vi "Resize Message String & Dialog Window.vi"(6 "Max Number of Lines":i32, 8 "Error In":errorcluster, 9 "Message":string, 10 "Controls & Indicators":T1, 11 "VI Refnum":refnum<vi>) -> (0 "Error Out":errorcluster, 3 "VI Refnum out":refnum<vi>)   [LabVIEW 2021, in "GUI.lvlib"]
uses:
  GUI.lvlib
  Error/Error.lvlib
  Buttons/Buttons.lvlib
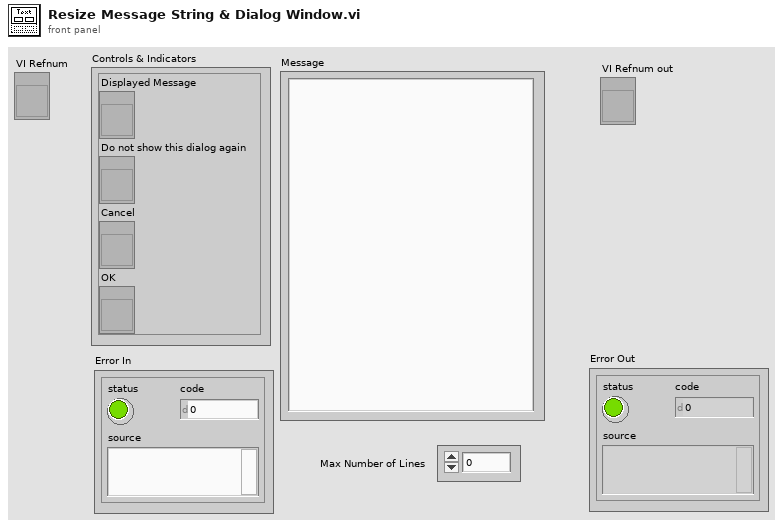
[diagram p1: front panel]
types:
  T1 = cluster{"Displayed Message":refnum<vi>, "Do not show this dialog again":refnum<vi>, "Cancel":refnum<vi>, "OK":refnum<vi>}
  T2 = typedef "LVRectTypeDef.ctl" = cluster{"Left":i16, "Top":i16, "Right":i16, "Bottom":i16}
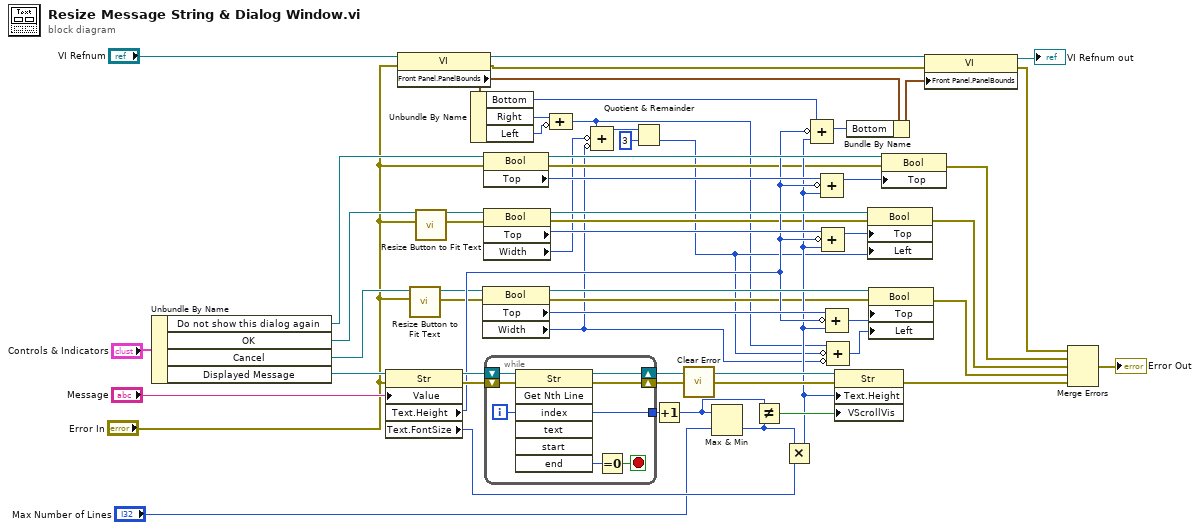
[diagram p0: block diagram]
diagram:
  n1 = Unbundle By Name("Controls & Indicators") -> ("Do not show this dialog again"=w37:refnum<vi>, "OK"=w9:refnum<vi>, "Cancel"=w33:refnum<vi>, "Displayed Message"=w44:refnum<vi>)
  n2 = property class="Str"(reference=w44, error in="Error In", "Value"="Message") -> (reference out=w58:refnum<vi>, error out=w57:errorcluster, "Text.Height"=w27:u32, "Text.FontSize"=w54:u32)
  n3 = property class="VI"(reference="VI Refnum", error in="Error In") -> (reference out=w40:refnum<vi>, error out=w39:errorcluster, "Front Panel.PanelBounds"=w42:T2)
  n4 = call "Resize Button to Fit Text.vi"("error in (no error)"="Error In", "Boolean in"=w33) -> ("error out"=w10:errorcluster, "Boolean out"=w11:refnum<vi>)  [unwired: 8 in]
  n5 = call "Resize Button to Fit Text.vi"("error in (no error)"="Error In", "Boolean in"=w9) -> ("error out"=w6:errorcluster, "Boolean out"=w8:refnum<vi>)  [unwired: 8 in]
  n6 = Unbundle By Name(w42) -> ("Bottom"=w43:i16, "Right"=w15:i16, "Left"=w14:i16)
  n7 = property class="Bool"(reference=w11, error in=w10) -> (reference out=w31:refnum<vi>, error out=w21:errorcluster, "Top"=w28:i32, "Width"=w17:u32)
  n8 = property class="Bool"(reference=w37, error in="Error In") -> (reference out=w35:refnum<vi>, error out=w23:errorcluster, "Top"=w36:i32)
  n9 = property class="Bool"(reference=w8, error in=w6) -> (reference out=w32:refnum<vi>, error out=w22:errorcluster, "Top"=w30:i32, "Width"=w20:u32)
  n10 = while {
    shift-right: [w64] -> w52
    shift-left: w57 -> [w65]
    shift-right: [w63] -> w53
    shift-left: w58 -> [w66]
    tunnel: [w61] -> w55
    i -> [w61]
    stop <- w60 stop-if-true
    n11 = invoke class="Str" method="Get Nth Line"(reference=w66, error in=w65, "index"=w61) -> (reference out=w63:refnum<vi>, error out=w64:errorcluster, "end"=w62:u32)  [unwired: 4 in, 4 out]
    n12 = Equal To 0?(x=w62) -> (x = 0?=w60:bool)
  }
  n13 = Compound Arithmetic op=ADD(w15, invert w14) -> (w13:i16)
  n14 = Compound Arithmetic op=ADD(w13, invert w20, invert w17) -> (w19:u32)
  n15 = Quotient & Remainder(x=w19, y=u32 3) -> (floor(x/y)=w16:u32)  [unwired: 1 out]
  n16 = Increment(x=w55) -> (x+1=w48:i32)
  n17 = call "Clear Error.vi"("Error In"=w52) -> ("no Error Out"=w50:errorcluster)  [unwired: 8 in]
  n18 = Max & Min(x=w48, y="Max Number of Lines") -> (min(x,y)=w49:i32)  [unwired: 1 out]
  n19 = Not Equal?(x=w48, y=w49) -> (x != y?=w47:bool)
  n20 = Multiply(x=w49, y=w54) -> (x*y=w26:u32)
  n21 = Compound Arithmetic op=ADD(w43, invert w27, w26) -> (w41:u32)
  n22 = Compound Arithmetic op=ADD(w36, invert w27, w26) -> (w34:u32)
  n23 = Compound Arithmetic op=ADD(w30, invert w27, w26) -> (w29:u32)
  n24 = Compound Arithmetic op=ADD(w28, invert w27, w26) -> (w25:u32)
  n25 = Compound Arithmetic op=ADD(w13, invert w16, invert w17) -> (w12:u32)
  n26 = property class="Str"(reference=w53, error in=w50, "Text.Height"=w26, "VScrollVis"=w47) -> (error out=w51:errorcluster)  [unwired: 1 out]
  n27 = Bundle By Name(cluster=w42, "Bottom"=w41) -> (w38:T2)
  n28 = property class="Bool"(reference=w32, error in=w22, "Top"=w29, "Left"=w16) -> (error out=w3:errorcluster)  [unwired: 1 out]
  n29 = property class="Bool"(reference=w31, error in=w21, "Top"=w25, "Left"=w12) -> (error out=w4:errorcluster)  [unwired: 1 out]
  n30 = property class="Bool"(reference=w35, error in=w23, "Top"=w34) -> (error out=w2:errorcluster)  [unwired: 1 out]
  n31 = property class="VI"(reference=w40, error in=w39, "Front Panel.PanelBounds"=w38) -> (reference out=→"VI Refnum out":refnum<vi>, error out=w1:errorcluster)
  n32 = Merge Errors(w1, w2, w3, w4, w51) -> (→"Error Out":errorcluster)
